vi "Create Text Objects.vi"(8 "error in (no error)":errorcluster, 10 "VI Name":string, 11 "Control In":refnum<class "Control.lvclass">) -> (0 "error out":errorcluster, 2 "JS Indicator":string, 3 "Control Out":refnum<class "Control.lvclass">, 5 "HTML":string)   [LabVIEW 2017, in "Front Panel Publisher.lvlib" / "Control.lvclass"]
uses:
  Control.lvclass
  Text_class/Text.lvclass
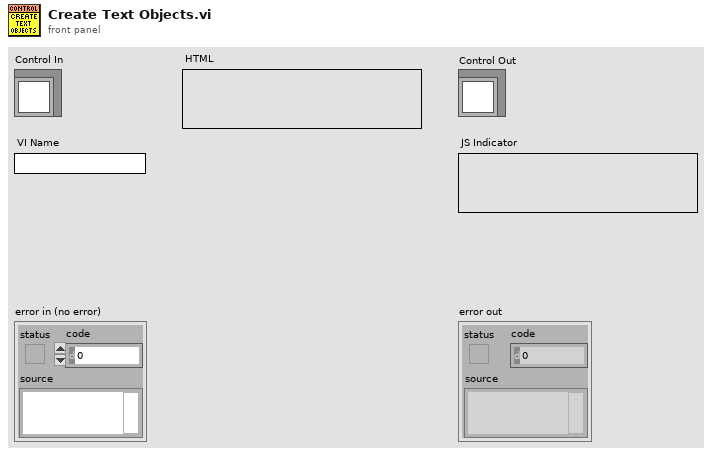
[diagram p1: front panel]
types:
  T1 = typedef "Front Panel Publisher.lvlib/Control.lvclass/Attributes.ctl" = cluster{"Description":string, "Indicator":bool, "Default Value":variant, "Control Index":i32, "Label":refnum<class "Text.lvclass">, "Caption":refnum<class "Text.lvclass">, "Image b64":string, "No Control Index":bool, "Display Mode":T2}
  T2 = typedef "Front Panel Publisher.lvlib/Web Front Panel.lvclass/Enum - Control Display Mode.ctl" = enum16{"Value Only", "Value and Visibility", "Boolean Value Only", "Boolean Value and Visibility", "Control is Image", "Image and Visibility"}
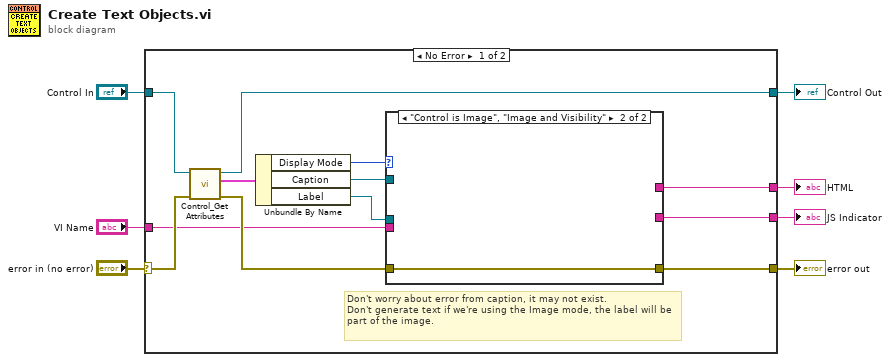
[diagram p0: block diagram]
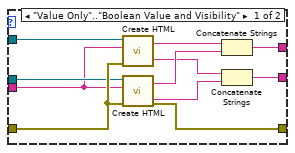
[diagram p2: hidden frame]
diagram:
  n1 = case shown="No Error" "error in (no error)" {
    selector: "error in (no error)" -> [w19 w33]
    tunnel: [w17 w33] -> w6
    tunnel: [w14 w32] -> w4
    tunnel: "Control In" -> [w15 w32]
    tunnel: [w11 _] -> w3
    tunnel: "VI Name" -> [w10 _]
    tunnel: [w8 _] -> w1
    frame No Error {
      # "Don't worry about error from caption, it may not exist.\nDon't generate text if we're using the Image mode, the label will be part of the image."
      n2 = call "Control_Get Attributes.vi"("error in (no error)"=w19, "Control In"=w15) -> ("error out"=w18:errorcluster, "Control Attributes"=w16:T1, "Control Out"=w14:refnum<class "Control.lvclass">)  [unwired: 7 in]
      n3 = Unbundle By Name(w16) -> ("Display Mode"=w9:T2, "Caption"=w13:refnum<class "Text.lvclass">, "Label"=w12:refnum<class "Text.lvclass">)
      n4 = case shown="\"Control is Image\", \"Image and Visibility\"" w9 {
        tunnel: w18 -> [w30 w31]
        tunnel: [w29 w31] -> w17
        tunnel: w13 -> [w28 _]
        tunnel: w12 -> [w27 _]
        tunnel: [w22 _] -> w11
        tunnel: w10 -> [w24 _]
        tunnel: [w20 _] -> w8
        frame "Value Only".."Boolean Value and Visibility" {
          n5 = call-dynamic "Create HTML.vi"("error in (no error)"=w30, "VI Identifier"=w24, "Text In"=w28) -> ("HTML"=w26:string, "js code for indicators"=w23:string)  [unwired: 2 in, 5 out]
          n6 = call-dynamic "Create HTML.vi"("error in (no error)"=w30, "VI Identifier"=w24, "Text In"=w27) -> ("error out"=w29:errorcluster, "HTML"=w25:string, "js code for indicators"=w21:string)  [unwired: 2 in, 4 out]
          n7 = Concatenate Strings(w26, w25) -> (w22:string)
          n8 = Concatenate Strings(w23, w21) -> (w20:string)
        }
        frame "Control is Image", "Image and Visibility" {
        }
      }
    }
    frame Error {
    }
  }
  "error out" <- w6
  "Control Out" <- w4
  "HTML" <- w3
  "JS Indicator" <- w1
